vi "Next_Field.vi"(7 "Field and Temp Array Controller":cluster{"Field (T)":dbl[], "Temps (K)":dbl[]}, 8 "error in (no error)":errorcluster, 9 "MagQ In":refnum<queue>, 10 "Temp and Field Range in":T2={"Temps(K)"=[], "Fields(T)"=[], "Sweep States"=enum."1. Idle", "PointStep"=enum."1. Scan_1", "Current Field"=0.0, "Current Temp"=0.0, "Expected_ACK"=enum."1. None", "ACK"=enum."1. None", "AfterAckStep"=enum."1. Idle", "Current Index Field"=0, "Current Index Temp"=0, "ACK Structure "=enum."Inner"}, 11 "Queue in":refnum<queue>) -> (0 "error out":errorcluster, 1 "MagQ Out":refnum<queue>, 2 "Temp and Field Range out":T2={"Temps(K)"=[], "Fields(T)"=[], "Sweep States"=enum."1. Idle", "PointStep"=enum."1. Scan_1", "Current Field"=0.0, "Current Temp"=0.0, "Expected_ACK"=enum."1. None", "ACK"=enum."1. None", "AfterAckStep"=enum."1. Idle", "Current Index Field"=0, "Current Index Temp"=0, "ACK Structure "=enum."Inner"}, 3 "Queue out":refnum<queue>, 4 "Field and Temp Array Controller 3":cluster{"Field (T)":dbl[], "Temps (K)":dbl[]}, 5 "PSU Status Out":T1={"Ramp Target"=enum."ZERO", "Pause"=FALSE, "Switch Heater"=FALSE, "Persistent Field"=0.0, "Persistent Current"=0.0, "Tesla"=FALSE, "Output (T)"=0.0, "Output (A)"=0.0, "X Trip"=enum."DISABLED", "Ramp Rate (A/s)"=0.0, "V Limit (V)"=0.0, "Heater Voltage"=0.0, "MAX Setpoint (A)"=0.0, "MAX Setpoint (T)"=0.0, "MID Setpoint (A)"=0.0, "MID Setpoint (T)"=0.0, "Lock"=FALSE, "Field Constant"=0.0, "Remote"=FALSE, "Direction"=enum."POSITIVE", "Helium Level"=0, "Quench !"=FALSE, "Voltage"=0.0, "V Limit !"=FALSE, "Ramping"=FALSE, "At Target"=FALSE, "Trip Field"=0.0, "Trip Current"=0.0, "Current State"=enum."1. INIT MAG", "MAG Reference"="COM4"} {"Trip Current" format="%.3f"; "Trip Field" format="%.4f"; "Voltage" format="%.2f"; "Field Constant" format="%.6f"; "MID Setpoint (T)" format="%.4f"; "MID Setpoint (A)" format="%.3f"; "MAX Setpoint (T)" format="%.4f"; "MAX Setpoint (A)" format="%.3f"; "Heater Voltage" format="%.2f"; "V Limit (V)" format="%.2f"; "Ramp Rate (A/s)" format="%.3f"; "Output (A)" format="%.3f"; "Output (T)" format="%.4f"; "Persistent Current" format="%.3f"; "Persistent Field" format="%.4f"})   [LabVIEW 2025]
uses:
  CTLS/Sweeper.ctl
  CTLS/PSU Status.ctl
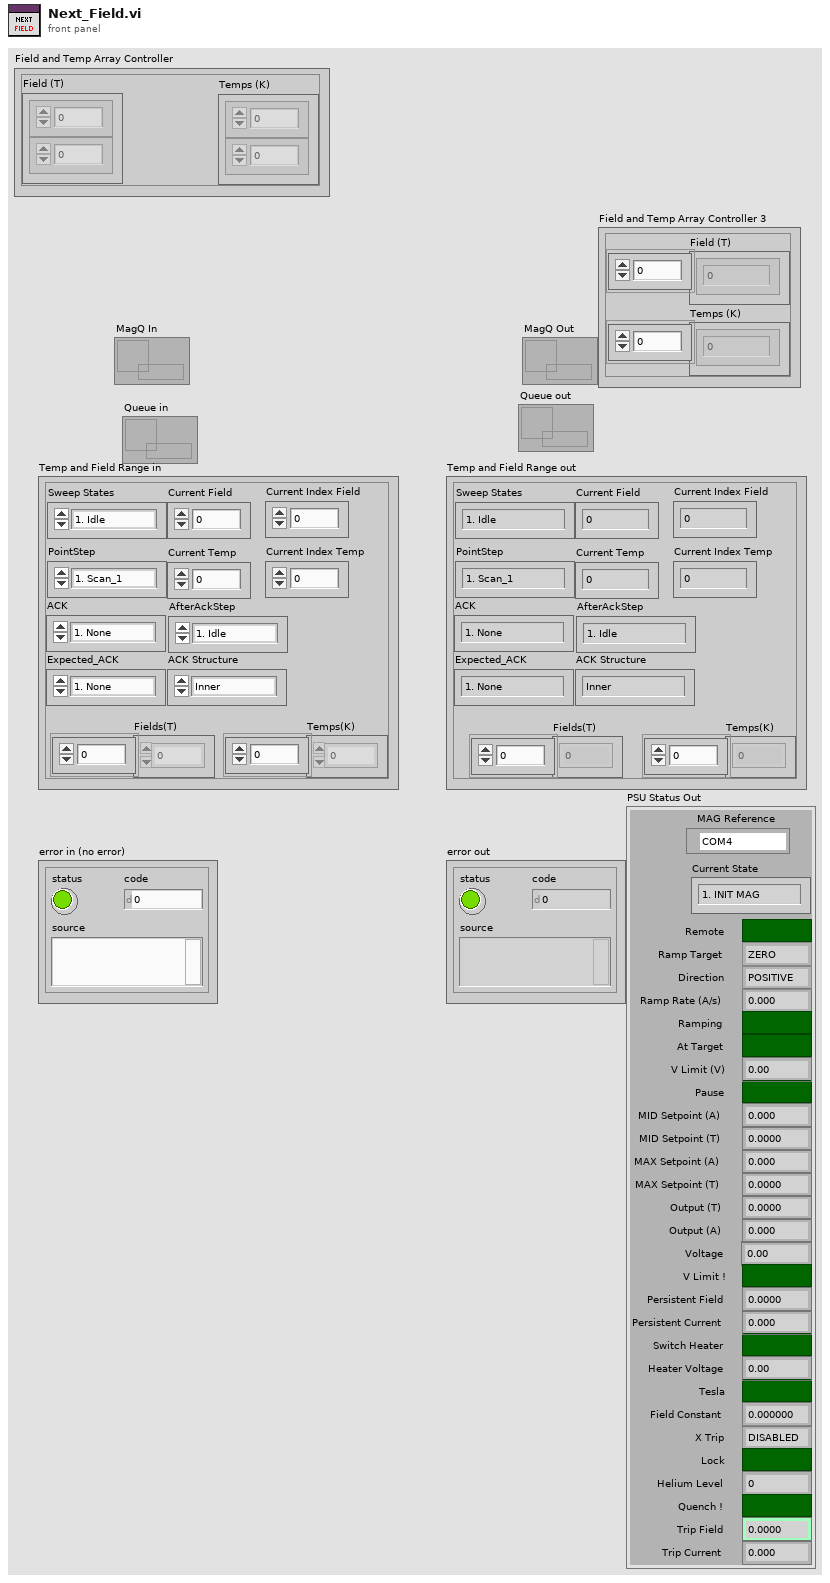
[diagram p1: front panel]
types:
  T1 = typedef "PSU Status.ctl" = cluster{"Ramp Target":enum16{"ZERO", "MID", "MAX"}, "Pause":bool, "Switch Heater":bool, "Persistent Field":dbl, "Persistent Current":dbl, "Tesla":bool, "Output (T)":dbl, "Output (A)":dbl, "X Trip":enum16{"DISABLED", "ENABLED", "ACTIVE"}, "Ramp Rate (A/s)":dbl, "V Limit (V)":dbl, "Heater Voltage":dbl, "MAX Setpoint (A)":dbl, "MAX Setpoint (T)":dbl, "MID Setpoint (A)":dbl, "MID Setpoint (T)":dbl, "Lock":bool, "Field Constant":dbl, "Remote":bool, "Direction":enum16{"POSITIVE", "NEGATIVE", "OPEN", "UNIPOLAR"}, "Helium Level":u16, "Quench !":bool, "Voltage":dbl, "V Limit !":bool, "Ramping":bool, "At Target":bool, "Trip Field":dbl, "Trip Current":dbl, "Current State":enum16{"1. INIT MAG", "2. MAG ON", "3. MAG_STAB", "4. MAG IDLE", "5. MAG OFF (Reset)"}, "MAG Reference":refnum<visa-resource-name>}
  T2 = typedef "Sweeper.ctl" = cluster{"Temps(K)":dbl[], "Fields(T)":dbl[], "Sweep States":enum16{"1. Idle", "2. Start", "3. Apply_Config", "4. Run_Point_Step", "5. Wait ACK", "6. Next Field", "7. Next Temp", "8. Stop"}, "PointStep":enum16{"1. Init_Bias", "2. Init_Scan", "3. Field_Stable", "4. Temp_stable", "1. Scan_1", "2. DC_SF_1", "3. DC_BS_1", "4. Bias", "5. Scan_2", "6. DC_SF_2", "7. DC_BS_2", "8. Done"}, "Current Field":dbl, "Current Temp":dbl, "Expected_ACK":enum16{"1. None", "2. TempStable", "3. FieldStable", "4. ConfigApplied", "5. ScanDone", "6. BiasDone", "7. DriftDone (SF)", "8. DrifDone (BS)", "9. Done"}, "ACK":enum16{"1. None", "2. TempStable", "3. FieldStable", "4. ConfigApplied", "5. ScanDone", "6. BiasDone", "7. DriftDone (SF)", "8. DrifDone (BS)", "9. Done"}, "AfterAckStep":enum16{"1. Idle", "2. Start", "3. Apply_Config", "4. Run_Point_Step", "5. Wait ACK", "6. Next Field", "7. Next Temp", "8. Stop"}, "Current Index Field":i32, "Current Index Temp":i32, "ACK Structure ":enum16{"Inner", "Outer"}}
  T3 = enum16{"1. Init_Bias", "2. Init_Scan", "3. Field_Stable", "4. Temp_stable", "1. Scan_1", "2. DC_SF_1", "3. DC_BS_1", "4. Bias", "5. Scan_2", "6. DC_SF_2", "7. DC_BS_2", "8. Done"}
  T4 = enum16{"1. Idle", "2. Start", "3. Apply_Config", "4. Run_Point_Step", "5. Wait ACK", "6. Next Field", "7. Next Temp", "8. Stop"}
  T5 = enum16{"1. None", "2. TempStable", "3. FieldStable", "4. ConfigApplied", "5. ScanDone", "6. BiasDone", "7. DriftDone (SF)", "8. DrifDone (BS)", "9. Done"}
  T6 = enum16{"1. INIT MAG", "2. MAG ON", "3. MAG_STAB", "4. MAG IDLE", "5. MAG OFF (Reset)"}
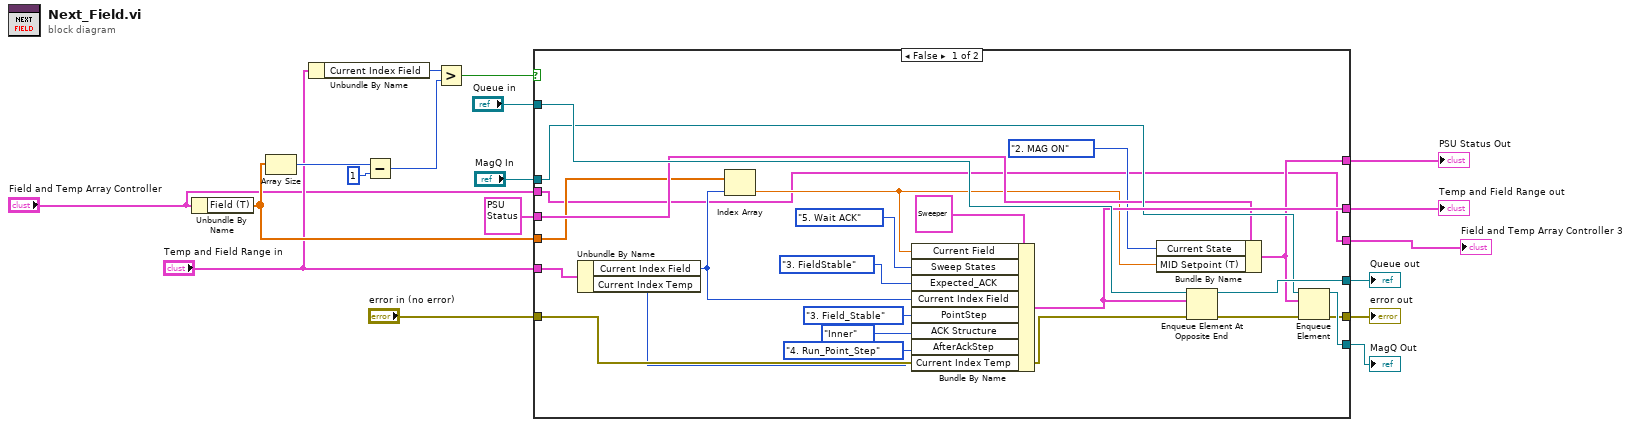
[diagram p0: block diagram]
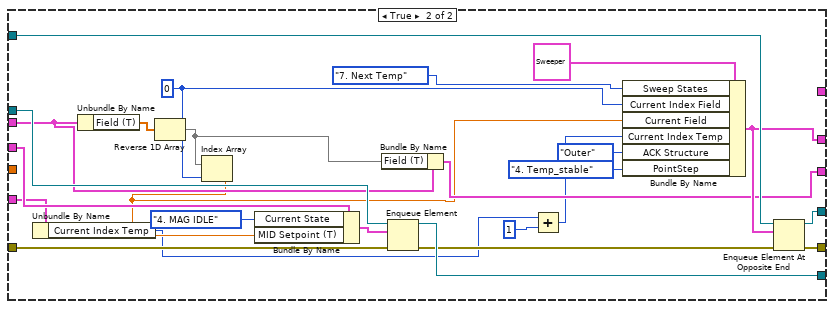
[diagram p2: hidden frame]
diagram:
  n1 = Unbundle By Name("Field and Temp Array Controller") -> ("Field (T)"=w4:dbl[])
  n2 = Array Size(array=w4) -> (size(s)=w11:i32)
  n3 = Unbundle By Name("Temp and Field Range in") -> ("Current Index Field"=w9:i32)
  n4 = Subtract(x=w11, y=1) -> (x-y=w12:i32)
  n5 = Greater?(x=w9, y=w12) -> (0:w10:bool)
  n6 = case shown="False" w10 {
    tunnel: [w37 w61] -> w14
    tunnel: "Queue in" -> [w41 w62]
    tunnel: [w39 w60] -> w16
    tunnel: [w29 w65] -> w17
    tunnel: "error in (no error)" -> [w40 w55]
    tunnel: "MagQ In" -> [w36 w57]
    tunnel: T1 {"Ramp Target"=enum."ZERO", "Pause"=FALSE, "Switch Heater"=FALSE, "Persistent Field"=0.0, "Persistent Current"=0.0, "Tesla"=FALSE, "Output (T)"=0.0, "Output (A)"=0.0, "X Trip"=enum."DISABLED", "Ramp Rate (A/s)"=0.0, "V Limit (V)"=0.0, "Heater Voltage"=0.0, "MAX Setpoint (A)"=0.0, "MAX Setpoint (T)"=0.0, "MID Setpoint (A)"=0.0, "MID Setpoint (T)"=0.0, "Lock"=FALSE, "Field Constant"=0.0, "Remote"=FALSE, "Direction"=enum."POSITIVE", "Helium Level"=0, "Quench !"=FALSE, "Voltage"=0.0, "V Limit !"=FALSE, "Ramping"=FALSE, "At Target"=FALSE, "Trip Field"=0.0, "Trip Current"=0.0, "Current State"=enum."1. INIT MAG", "MAG Reference"="COM4"} ("PSU Status In") -> [w33 w59]
    tunnel: [w35 w56] -> w7
    tunnel: [w30 _] -> w6
    tunnel: w4 -> [w28 _]
    tunnel: "Field and Temp Array Controller" -> [w21 w52]
    tunnel: "Temp and Field Range in" -> [w27 w47]
    tunnel: [w21 w51] -> w1
    frame False {
      n7 = Unbundle By Name(w27) -> ("Current Index Field"=w24:i32, "Current Index Temp"=w19:i32)
      n8 = Index Array(array=w28, index=w24) -> (element=w31:dbl)
      n9 = Bundle By Name(cluster=T2 {"Temps(K)"=[], "Fields(T)"=[], "Sweep States"=enum."1. Idle", "PointStep"=enum."1. Scan_1", "Current Field"=0.0, "Current Temp"=0.0, "Expected_ACK"=enum."1. None", "ACK"=enum."1. None", "AfterAckStep"=enum."1. Idle", "Current Index Field"=0, "Current Index Temp"=0, "ACK Structure "=enum."Inner"} ("Temp and Field Range"), "Current Field"=w31, "Sweep States"=T4."5. Wait ACK", "Expected_ACK"=T5."3. FieldStable", "Current Index Field"=w24, "PointStep"=T3."3. Field_Stable", "ACK Structure"=enum16{"Inner", "Outer"}."Inner", "AfterAckStep"=T4."4. Run_Point_Step", "Current Index Temp"=w19) -> (w37:T2)
      n10 = Bundle By Name(cluster=w33, "Current State"=T6."2. MAG ON", "MID Setpoint (T)"=w31) -> (w30:T1)
      n11 = Enqueue Element At Opposite End(queue=w41, element=w37, error in (no error)=w40) -> (queue out=w39:refnum<queue>, error out=w34:errorcluster)  [unwired: 1 in, 1 out]
      n12 = Enqueue Element(queue=w36, element=w30, error in (no error)=w34) -> (queue out=w35:refnum<queue>, error out=w29:errorcluster)  [unwired: 1 in, 1 out]
    }
    frame True {
      w63 = 0 ("Current Index Field")
      n13 = Unbundle By Name(w47) -> ("Current Index Temp"=w46:i32)
      n14 = Unbundle By Name(w52) -> ("Field (T)"=w50:dbl[])
      n15 = Reverse 1D Array(array=w50) -> (reversed array=w49:dbl[])
      n16 = Index Array(array=w49, index=w63) -> (element=w48:dbl)
      n17 = Bundle By Name(cluster=w59, "Current State"=T6."4. MAG IDLE", "MID Setpoint (T)"=w48) -> (w58:T1)
      n18 = Bundle By Name(cluster=w52, "Field (T)"=w49) -> (w51:cluster{"Field (T)":dbl[], "Temps (K)":dbl[]})
      n19 = Enqueue Element(queue=w57, element=w58, error in (no error)=w55) -> (queue out=w56:refnum<queue>, error out=w54:errorcluster)  [unwired: 1 in, 1 out]
      n20 = Add(x=w46, y=1) -> (x+y=w44:i32)
      n21 = Bundle By Name(cluster=T2 {"Temps(K)"=[], "Fields(T)"=[], "Sweep States"=enum."1. Idle", "PointStep"=enum."1. Scan_1", "Current Field"=0.0, "Current Temp"=0.0, "Expected_ACK"=enum."1. None", "ACK"=enum."1. None", "AfterAckStep"=enum."1. Idle", "Current Index Field"=0, "Current Index Temp"=0, "ACK Structure "=enum."Inner"} ("Temp and Field Range"), "Sweep States"=T4."7. Next Temp", "Current Index Field"=w63, "Current Field"=w48, "Current Index Temp"=w44, "ACK Structure"=enum16{"Inner", "Outer"}."Outer", "PointStep"=T3."4. Temp_stable") -> (w61:T2)
      n22 = Enqueue Element At Opposite End(queue=w62, element=w61, error in (no error)=w54) -> (queue out=w60:refnum<queue>, error out=w65:errorcluster)  [unwired: 1 in, 1 out]
    }
  }
  "error out" <- w17
  "Queue out" <- w16
  "Temp and Field Range out" <- w14
  "MagQ Out" <- w7
  "PSU Status Out" <- w6
  "Field and Temp Array Controller 3" <- w1
